vi "TCP Close connection.vi"(8 "error in (no error)":errorcluster, 10 "abort (F)":bool, 11 "TCP in":refnum<class "TCP.lvclass">) -> (0 "error out":errorcluster, 3 "TCP out":refnum<class "TCP.lvclass">)   [LabVIEW 2013, in "TCP.lvclass"]
doc: "Closes a TCP network connection"
uses:
  TCP.lvclass
  TCP.lvclass/TCP.ctl
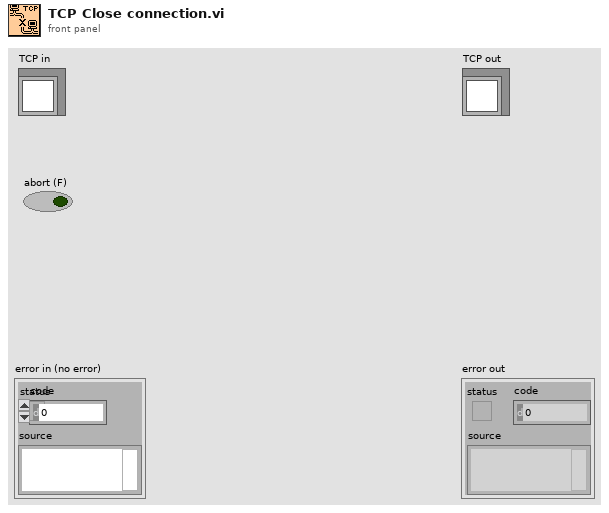
[diagram p1: front panel]
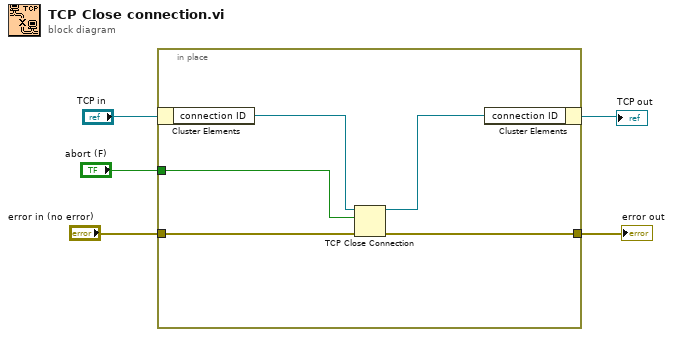
[diagram p0: block diagram]
diagram:
  n1 = in-place {
    in-place-border: "error in (no error)" -> [w8]
    in-place-border: [w7] -> w2
    in-place-border: "abort (F)" -> [w6]
    n2 = in-place-cluster #1("TCP in") -> ("connection ID"=w10:refnum<k5>)
    n3 = TCP Close Connection(connection ID=w10, abort (F)=w6, error in (no error)=w8) -> (connection ID out=w9:refnum<k5>, error out=w7:errorcluster)
    n4 = in-place-cluster #1("connection ID"=w9) -> (→"TCP out":refnum<class "TCP.lvclass">)
  }
  "error out" <- w2
